vi "SimEx Writing Model Parameters to RT.vi"   [LabVIEW 2011]
doc: "This example shows how to use the Read/Write Model Parameters function to change the values of model parameters in a simulation hierarchy that is running on an RT target."
uses:
  <vilib>/Simulation/Param Hierarchy/ParamBlockSupport/SIMPH Read or Write Mode.ctl
  Read-Write Model Parameters/subVIs/subsystem with sine wave.vi
  <vilib>/Simulation/Param Hierarchy/ParamBlockSupport/SIMPH Reset Call Chain.vi
  <vilib>/Simulation/Param Hierarchy/SIMPH Read Simulation Parameter.vi
  <vilib>/Simulation/Param Hierarchy/SIMPH Write Simulation Parameter.vi
  <vilib>/Simulation/Param Hierarchy/ParamBlock/SIMPH_ParamBlock.xnode
panel:
  # "See Block Diagram"
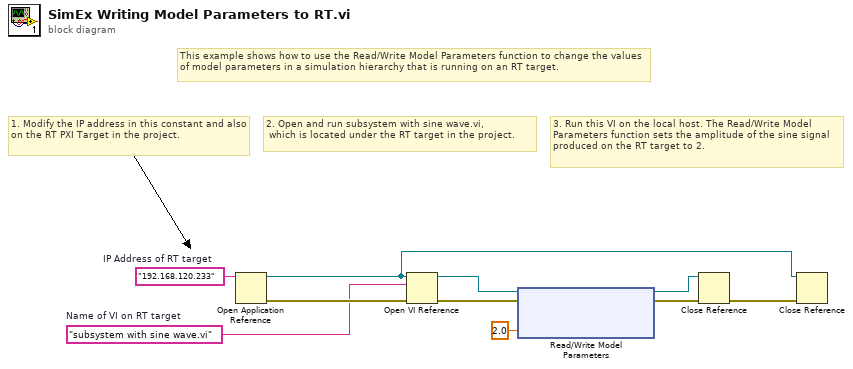
[diagram p0: block diagram]
diagram:
  w2 = "subsystem with sine wave.vi"  # Name of VI on RT target
  w7 = "192.168.120.233"  # IP Address of RT target
  # "This example shows how to use the Read/Write Model Parameters function to change the values of model parameters in a simulation hierarchy that is running on an RT target."
  # "2. Open and run subsystem with sine wave.vi,\n which is located under the RT target in the project."
  # "1. Modify the IP address in this constant and also on the RT PXI Target in the project."
  # "3. Run this VI on the local host. The Read/Write Model Parameters function sets the amplitude of the sine signal produced on the RT target to 2."
  n1 = Open Application Reference(11:w7) -> (0:w8:errorcluster, 3:w3:refnum<vi>)  [unwired: 3 in]
  n2 = Open VI Reference(application reference (local)=w3, vi path=w2, error in (no error)=w8) -> (vi reference=w9:refnum<vi>, error out=w10:errorcluster)  [unwired: 3 in]
  n3 = xnode "Read/Write Model Parameters"("VI reference in"=w9, "error in"=w10, "value"=2.0) -> ("VI reference out"=w4:refnum<vi>, "error out"=w6:errorcluster)
  n4 = Close Reference(reference=w4, error in (no error)=w6) -> (error out=w5:errorcluster)
  n5 = Close Reference(reference=w3, error in (no error)=w5) -> ()  [unwired: 1 out]
